vi "is_done.vi"(8 "error in (no error)":errorcluster, 11 "Counter in":refnum<class "Counter.lvclass">) -> (0 "error out":errorcluster, 2 "task done?":bool, 3 "Counter out":refnum<class "Counter.lvclass">)   [LabVIEW 2014, in "Counter.lvclass"]
uses:
  Counter.lvclass
  Counter.lvclass/Counter.ctl
  Globals.vi
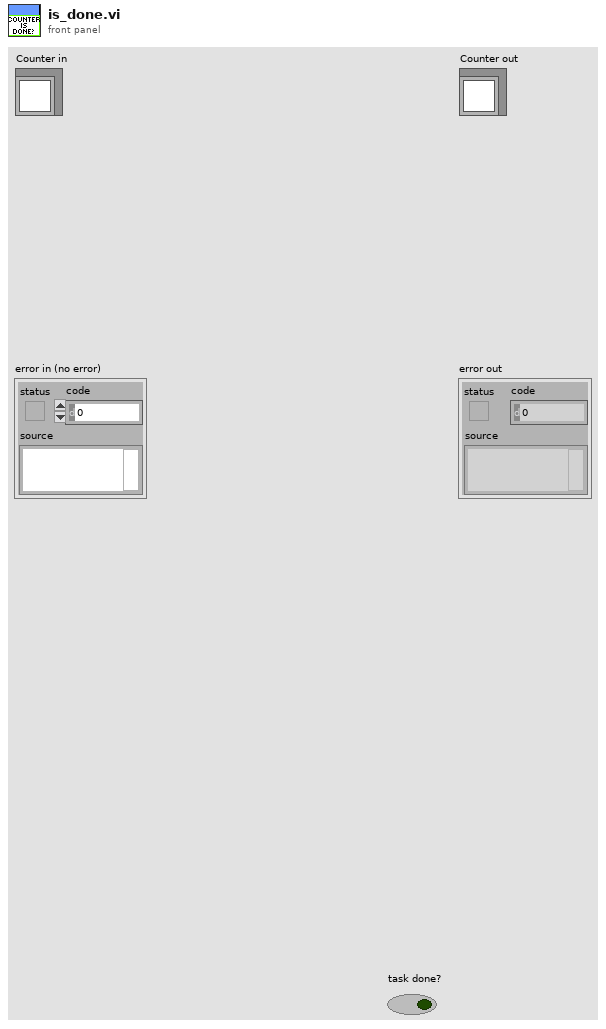
[diagram p1: front panel]
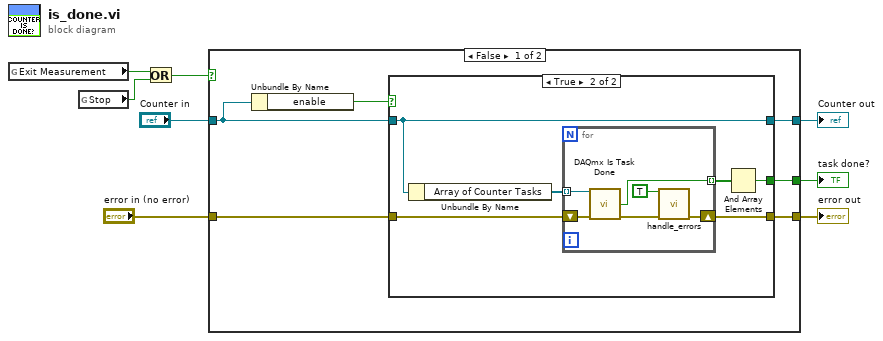
[diagram p0: block diagram]
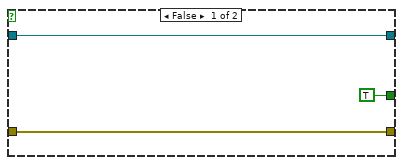
[diagram p2: hidden frame]
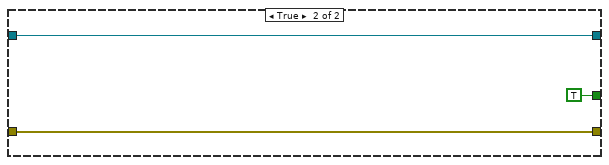
[diagram p3: hidden frame]
diagram:
  n1 = global read "Globals.vi" "Exit Measurement"() -> (w8:bool)
  n2 = global read "Globals.vi" "Stop"() -> (w7:bool)
  n3 = Or(x=w8, y=w7) -> (x .or. y?=w6:bool)
  n4 = case shown="False" w6 {
    tunnel: [w13 w31] -> w1
    tunnel: [w9 w32] -> w3
    tunnel: "Counter in" -> [w10 w32]
    tunnel: "error in (no error)" -> [w12 w31]
    tunnel: [w11 TRUE ("Exit Measurement")] -> w5
    frame False {
      n5 = Unbundle By Name(w10) -> ("enable"=w14:bool)
      n6 = case shown="True" w14 {
        tunnel: w12 -> [w17 w21]
        tunnel: [w17 w18] -> w13
        tunnel: [TRUE ("task done?") w19] -> w11
        tunnel: w10 -> [w15 w23]
        tunnel: [w15 w23] -> w9
        frame False {
        }
        frame True {
          n7 = Unbundle By Name(w23) -> ("Array of Counter Tasks"=w22:refnum<k21>[])
          n8 = for {
            tunnel: w22 -> [w29] mode=indexing
            shift-right: [w26] -> w18
            shift-left: w21 -> [w28]
            tunnel: [w24] -> w20 mode=indexing
            n9 = call <vilib>:"DAQmx Is Task Done.vi"("task/channels in"=w29, "error in"=w28) -> ("task done?"=w24:bool, "error out"=w27:errorcluster)  [unwired: 11 in, 1 out]
            n10 = call "handle_errors.vi"("Exit Operation"=TRUE ("Exit Measurement"), "error in (no error)"=w27) -> ("error out"=w26:errorcluster)  [unwired: 13 in]
          }
          n11 = And Array Elements(Boolean array=w20) -> (logical AND=w19:bool)
        }
      }
    }
    frame True {
    }
  }
  "error out" <- w1
  "Counter out" <- w3
  "task done?" <- w5
